vi "Set Items in Device List.vi"(8 "Error In":errorcluster, 11 "Device List State":T1) -> (0 "Error Out":errorcluster, 3 "Device List State out":T1)   [LabVIEW 2015]
uses:
  Device List State.ctl
  Device/Device.lvclass
  Device/Read Name.vi
panel:
  in  "Menu Ring":u16(ring) items=["NONE", "Test class", "Device 1", "NI Lock-in", "Digitizer_1", "NI-DAQ dev1", "NI-DAQ dev2", "NI-DAQ extra"]
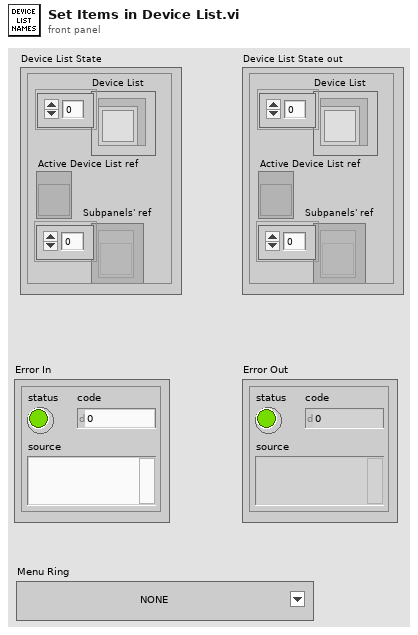
[diagram p1: front panel]
types:
  T1 = typedef "Device List State.ctl" = cluster{"Device List":refnum<class "Device.lvclass">[], "Active Device List ref":refnum<vi>, "Subpanels' ref":refnum<vi>[]}
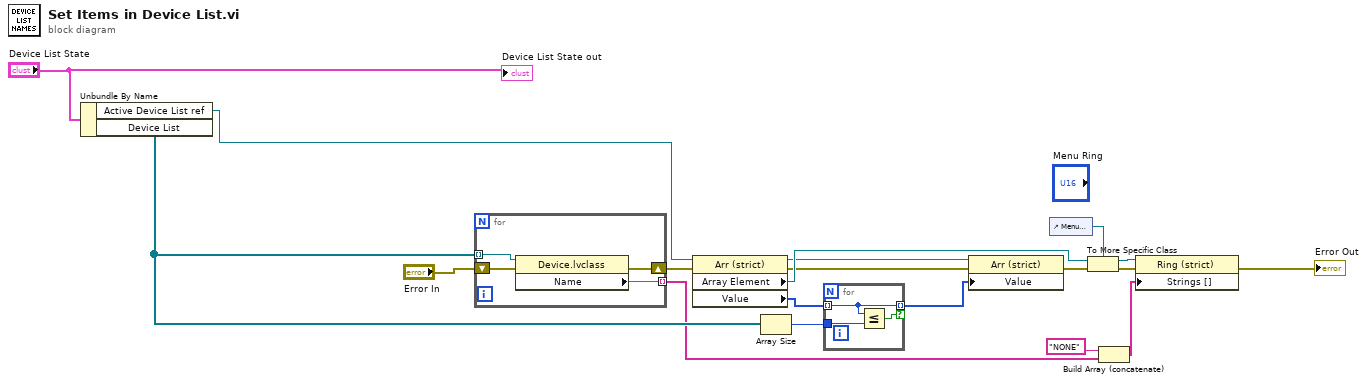
[diagram p0: block diagram]
diagram:
  n1 = Unbundle By Name("Device List State") -> ("Active Device List ref"=w17:refnum<vi>, "Device List"=w15:refnum<class "Device.lvclass">[])
  n2 = for {
    tunnel: w15 -> [w20] mode=indexing
    tunnel: [w21] -> w9 mode=indexing
    shift-right: [w23] -> w8
    shift-left: "Error In" -> [w22]
    n3 = property class="Device.lvclass"(reference=w20, error in=w22) -> (error out=w23:errorcluster, "Name"=w21:string)  [unwired: 1 out]
  }
  n4 = property class="Arr (strict)"(reference=w17, error in=w8) -> (reference out=w2:refnum<vi>, error out=w7:errorcluster, "Array Element"=w13:refnum<vi>, "Value"=w4:u16[])
  n5 = Array Size(array=w15) -> (size(s)=w14:i32)
  n6 = for {
    tunnel: w4 -> [w25] mode=indexing
    tunnel: w14 -> [w24]
    tunnel: [w25] -> w1 mode=indexing if=w26
    n7 = Less Or Equal?(x=w25, y=w24) -> (x <= y?=w26:bool)
  }
  n8 = property class="Arr (strict)"(reference=w2, error in=w7, "Value"=w1) -> (error out=w3:errorcluster)  [unwired: 1 out]
  n9 = control-ref of="Menu Ring"() -> (w5:refnum<vi>)
  n10 = To More Specific Class(target class=w5, reference=w13, error in=w3) -> (specific class reference=w12:refnum<vi>, error out=w6:errorcluster)
  n11 = Build Array (concatenate)("NONE", w9) -> (w10:string[])
  n12 = property class="Ring (strict)"(reference=w12, error in=w6, "Strings []"=w10) -> (error out=→"Error Out":errorcluster)  [unwired: 1 out]
  "Device List State out" <- "Device List State"
